vi "AlliGator Source Image Context Menu Handler.vi"(8 "Error In":errorcluster, 11 "Image Event Data":T3) -> (0 "Error Out":errorcluster, 3 "AlliGator Actions":T1[](array[typedef]))   [LabVIEW 2021, in "AlliGator Source Image.lvlib"]
doc: "Converts menu items into Source Image actions."
uses:
  AlliGator Source Image.lvlib
  Image/Image Display Event.ctl
  Image/Image Control Refnum.ctl
  <vilib>/Utility/miscctls.llb/LVPoint32TypeDef.ctl
  AlliGator Q Element.ctl
  AlliGator Q Event.ctl
  Image/Image Display to Clipboard Options.ctl
  AlliGator ROI Manager Actions.ctl
  AlliGator Selected ROI.ctl
  Image/Image Control ROI Description.ctl
  AlliGator Source Image ROI Manager.vi
  AlliGator Action Engine.lvlib
  Image/Image.lvlib
  Utilities/Utilities.lvlib
  AlliGator ROIs.lvlib
panel:
  # "see the AlliGator License on the block diagram (Ctrl+E or Window:Show Block Diagram)"
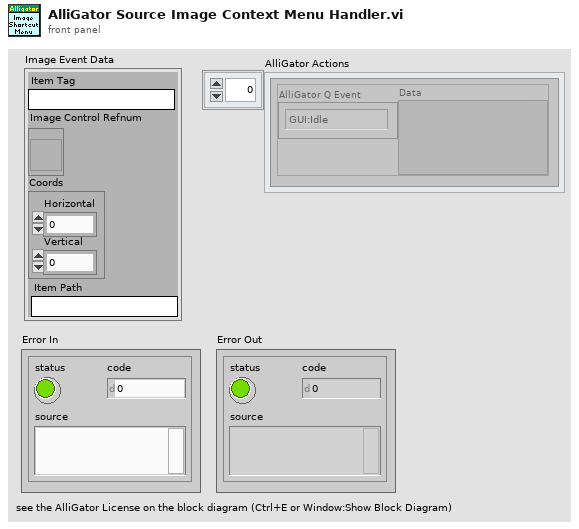
[diagram p1: front panel]
types:
  T1 = typedef "AlliGator Action Engine.lvlib/AlliGator Q Element.ctl" = cluster{"AlliGator Q Event":T2, "Data":variant}
  T2 = typedef "AlliGator Action Engine.lvlib/AlliGator Q Event.ctl" = enum16{"---- Files ----", "Files:Set Batch Export Files To Save", "Files:Set Dataset Loading & Pre-processing Options", "Files:Check #Frames in Dataset", "Files:Increment Frame Index", "Files:Open Mask Image", "Files:Open White Light Image", "Files:Open Single Dataset", "Files:New Folder of Folders Selected", "Files:Load File (all Types)_Scriptable", "Files:Move Flattened Series to Folders Series", "Files:Select Folder", "Files:Load FLI Dataset", "Files:Load Swiss SPAD 1 Dataset", "Files:Load Swiss SPAD 2 Dataset", "Files:Load .sdt FLI Dataset", "Files:Load .ptu FLI Dataset", "Files:Load .bin FLI Dataset", "Files:Load Single Gate Image Folder", "Files:Load I/m/phi Dataset (deprecated)", "Files:Load Single Image", "Files:Subtract Background File", "Files:Export FLI Dataset", "Files:Load HDF5 FLI Dataset", "Files:Set Destination File Path", "Files:Save Mask Image", "Files:Batch Conversion", "Files:New Folder Selected", "Files:Close FLI Dataset", "Files:Close FLI Dataset Series", "Files:Close White Light Image", "Files:Close Mask Image", "---- FLI Dataset ----", "FLI Dataset:Channel Arithmetic", "FLI Dataset:Export Average Lifetime Map as ASCII", "FLI Dataset:Export User-Defined Quantity Map as ASCII", "FLI Dataset:Python Function FLI Dataset Event", "FLI Dataset:ROI Analysis", "FLI Dataset:Tilted Logistic Square Gated IRF Characteristics Map", "FLI Dataset:Logistic Square Gated IRF Characteristics Map", "FLI Dataset:Square Gated IRF Characteristics Map", "FLI Dataset:Multi-ROI Single-Pixel Phasor Analysis", "FLI Dataset:Multi-ROI Single-Pixel NLSF Analysis", "FLI Dataset:All ROIs IRF Extraction", "FLI Dataset:All ROIs Decay Fit Non-Interactive (Fast + Individual IRF)", "FLI Dataset:All ROIs Phasor Analysis", "FLI Dataset:All ROIs Decay Fit", "FLI Dataset:Fluorescence Decay Statistics", "FLI Dataset:Update Decay Statistics Graph", "FLI Dataset:Get Decay from ROI", "FLI Dataset:All ROIs Average Lifetimes", "---- FLI Dataset Series ----", "FLI Dataset Series:Sum All Datasets in Series", "FLI Dataset Series:Add Dataset to Accumulated Dataset", "FLI Dataset Series:Display Accumulated Dataset", "FLI Dataset Series:Clear Dataset Series Sum", "FLI Dataset Series:Time-Series Analysis (NLSF)", "FLI Dataset Series:Time-Series Analysis (Phasor)", "---- Image ----", "Image:Update Image Profile Plots", "Image:Image Histogram Cursor Move", "Image:Image Histogram", "Image:Image Contrast", "Image:Set Image Histogram Cursor Move Flag", "Image:Clear Image Overlay", "Image:Use ROI as Search Area", "Image:Set ROI Diameter", "Image:Save Image Data as TIFF", "Image:Save Displayed Image with Overlay", "Image:Save Image Overlay Only", "Image:Save Image as Hot Pixel Mask", "Image:Change Source Image Color Palette", "Image:Copy Image to Clipboard", "Image:Source Image ROI Selection", "Image:Delete All ROIs", "Image:Delete All Unselected ROIs", "Image:Delete ROI", "Image:Merge All ROIs", "Image:Store ROI", "Image:Source Image ROI Storage", "Image:Export ROI Description to Notebook", "Image:Save ROI", "Image:Load ROI", "Image:Paste ROI Definition", "Image:Clear ROI", "Image:Identify ROIs in Mask Image", "Image:Create Complementary ROI", "Image:Create Contour ROI", "Image:Create ROI(s) from Pixels with Peak above Min_Scriptable", "Image:Create ROI(s) from Pixels with Intensity above Min_Scriptable", "Image:Compute ROI Statistics", "Image:Delete ROI(s) based on ROI Characteristics", "Image:Create ROI Grid", "Image:ROI to Individual Pixel ROIs", "Image:Python Function Source Image Event", "Image:Show Phasor Calibration Map ROI Centers", "Image:Convert ROI to Mask Image", "Image:Mouse Move", "Image:Mouse Up", "Image:Set Source Image Mouse Move Flag", "Image:Add Scale Bar Overlay", "Image:Delete Existing ROIs Option", "---- Decay ----", "Decay:Clear IRF/Reference Plot", "Decay:Clear Local IRFs", "Decay:Add Decay to Graph", "Decay:Smoothen Plot", "Decay:Smoothen Plot Tail", "Decay:Average Selected Plots", "Decay:Extract IRF", "Decay:Optimal IRF Extraction", "Decay:Threshold IRF", "Decay:Fit to Model IRF", "Decay:Fit IRF to Square Gate", "Decay:Fit IRF to Logistic Square Gate", "Decay:Fit IRF to Tilted Logistic Square Gate", "Decay:Create Bounding Cursors Set", "Decay:Export Bounding Cursors Definition to Notebook", "Decay:Denoise Plot", "Decay:Compute Cumulative Function", "Decay:Use as Reference Decay", "Decay:Show Reference Decay/IRF", "Decay:Extrapolate Decay", "Decay:Create Head & Tail Bounding Cursors", "Decay:Store Cursor-defined Head & Tail Fractions", "Decay:Rebin Plot", "Decay:1-Normalize Decay", "Decay:[0-1]-Normalize Plot", "Decay:Straighten Decay", "Decay:Shift Decay", "Decay:Fold Decay", "Decay:Fit Decay", "Decay:Global Fit of Selected Decays", "Decay:Post Global Fit Script", "Decay:Add Global Fit Parameters to Graph", "Decay:Add Decay Parameter(s) to Plot (Graph)", "Decay:Export Decay to Phasor Graph", "Decay:Plot Decay Shifts", "Decay:Compute Average Lifetime", "Decay:Plot Convolution", "Decay:Graph Tip Strip Update", "---- Decay Statistics ----", "Decay Statistics:Tip Strip Update", "---- Intensity Time Trace ----", "Intensity Time Trace:Use File Timestamp", "Intensity Time Trace:Load Intensity Corrections File", "Intensity Time Trace:Clear Intensity Corrections File", "Intensity Time Trace:Tip Strip Update", "---- Phasor Plot ----", "Phasor Plot:Build Phasor Plot", "Phasor Plot:Change Phasor Plot Color Palette", "Phasor Plot:Adjust Phasor Plot Display Range", "Phasor Plot:Highlight Image ROI in Phasor Plot", "Phasor Plot:Save Phasor Plot Image with Overlay", "Phasor Plot:Export Complex Phasor Map", "Phasor Plot:Export Phasor Ratio Map", "Phasor Plot:Export Average Lifetime Map", "Phasor Plot:Compute Phase Lifetime Histogram", "Phasor Plot:Compute Phasor Ratio Histogram", "Phasor Plot:Compute Phase Lifetime vs Intensity Scatter Plot", "Phasor Plot:Weber 2-Component Decomposition", "Phasor Plot:Update Phasor Color Map Vertices", "Phasor Plot:Clear Phasor Overlay", "Phasor Plot:Use Segment Extremities as References", "Phasor Plot:Use UC/Segment Intersections as References", "Phasor Plot:Use UC/Principal Axis Intersections as References", "Phasor Plot:Use UC/Linear Fit Intersections as References", "Phasor Plot:Update Phasor Plot Reference", "Phasor Plot:Show Local Phasor Info in Phasor Plot", "Phasor Plot:Update Phasor Plot State", "Phasor Plot:Phasor Plot ROI Storage", "Phasor Plot:Phasor Plot ROI Selection", "Phasor Plot:Python Function Phasor Plot Event", "Phasor Plot:Overlay Phasor ROI, Ratio or Map in Source Image", "Phasor Plot:Compute Decay of Selected Phasors", "Phasor Plot:Phasor at Image Pixel", "Phasor Plot:Mouse Move", "Phasor Plot:Mouse Up", "Phasor Plot:Display Range Mouse Move", "Phasor Plot:Set Mouse Move Flag", "---- Phasor Graph ----", "Phasor Graph:Calibrated Phasor Map Series", "Phasor Graph:Whole Image Phasor Scatter Plot (Todo)", "Phasor Graph:Get Phasor Value", "Phasor Graph:Create New Phasor Plot Dialog", "Phasor Graph:Update Last Phasor Value", "Phasor Graph:Update Phasor (m, phi)", "Phasor Graph:Remove Single Phasor from Plot", "Phasor Graph:Add Single Phasor to Plot", "Phasor Graph:Remove Phasor Plot", "Phasor Graph:Remove Selected Phasor Plots", "Phasor Graph:Clear Phasor Data", "Phasor Graph:Clear Phasor Graph", "Phasor Graph:Cursor Move", "Phasor Graph:Draw Cursor Connecting Line", "Phasor Graph:Clear Cursor Connecting Line", "Phasor Graph:Find UC Intersection", "Phasor Graph:Use UC/Cursor-Defined Line Intersections", "Phasor Graph:Use Selected Plots Fitted Line/UC Intersections", "Phasor Graph:Use Selected Plots Principal Axis/UC Intersections", "Phasor Graph:Show Single Phasor", "Phasor Graph:Save Single Phasor Plot", "Phasor Graph:Save All Phasor Plots", "Phasor Graph:Load Phasor Plot(s)", "Phasor Graph:Phasor Multiplication", "Phasor Graph:Compute Average Phasor", "Phasor Graph:Compute Multiple Average Phasors (Selected Plots)", "Phasor Graph:Export Single Phasor Plot Phase Lifetimes", "Phasor Graph:Phase Lifetime Trajectory", "Phasor Graph:Phase Lifetime vs Intensity Scatter Plot (deprecated)", "Phasor Graph:Parameter 2 vs Parameter 1 Scatter Plot", "Phasor Graph:Use Cursor n Location", "Phasor Graph:Set Reference n to Current Phase Lifetime Value", "Phasor Graph:Set Reference n to Lifetime Value", "Phasor Graph:Set Cursor n Location", "Phasor Graph:Save Phasor Graph Image", "Phasor Graph:Update SEPL Plot", "Phasor Graph:Export Single Phasor Plot Data", "Phasor Graph:Export Selected Phasor Plots Data", "Phasor Graph:Python Function Phasor Graph Event", "Phasor Graph:Tip Strip Update", "---- Calibration ----", "Calibration:Set Calibration Type", "Calibration:Load/Save Phasor Calibration", "Calibration:Load/Save Phasor Calibration Series", "Calibration:Load/Save Phasor Calibration Map", "Calibration:Use as Calibration", "Calibration:Compute Optimal Calibration from Phasor References", "Calibration:Clear Phasor Calibration", "Calibration:Use as Calibration Series", "Calibration:Use as Calibration Map", "Calibration:Clear Calibration Series", "Calibration:Clear Calibration Map", "Calibration:Apply Phasor Calibration", "Calibration:Update Single Plot Calibration", "Calibration:Update Multiple Plots Calibration", "Calibration:Clear Single Plot Calibration", "Calibration:Clear All Plots Calibrations", "Calibration:Clear Plot(s) Calibration(s)?", "Calibration:Phasor Calibration Maps (# Gates Series)", "---- Phasor Ratio ----", "Phasor Ratio:Clear Reference n", "Phasor Ratio:Toggle Selected Plot(s)  Lock to Reference 1", "Phasor Ratio:Use as Reference n", "Phasor Ratio:Send Reference n to Notebook", "Phasor Ratio:Toggle Selected Plot(s)  Lock to Reference 2", "Phasor Ratio:Compute Phasor Ratio at Mouse Location", "Phasor Ratio:Compute Phasor Plot's Average Phasor Ratio", "Phasor Ratio:Compute Time-Series Phasor Ratios", "Phasor Ratio:Fit Line to Phasor Ratio Plot", "Phasor Ratio:Save References", "Phasor Ratio:Load References", "Phasor Ratio:Update Phasor Reference 1", "Phasor Ratio:Update Phasor Reference 2", "Phasor Ratio:Move Cursor n to Reference n", "Phasor Ratio:Use as Phasor Reference 1 Lifetime", "Phasor Ratio:Use as Phasor Reference 2 Lifetime", "Phasor Ratio:Export Phasor Ratio Map as ASCII", "Phasor Ratio:Tip Strip Update", "---- Lifetime & Other Parameters Graph ----", "Lifetime:Tip Strip Update", "---- Decay Fit Parameter Map ----", "Decay Fit Parameter Map:Export ROI NLSF Data as ASCII", "Decay Fit Parameter Map:Set Decay Fit  Parameter Map Selection", "Decay Fit Parameter Map:Build Decay Fit Parameter Map", "Decay Fit Parameter Map:Change Decay Fit Parameter Map Color Palette", "Decay Fit Parameter Map:Export Decay Fit Parameter Map Data as ASCII", "Decay Fit Parameter Map:Export All Decay Fit Parameter Maps Data as ASCII", "Decay Fit Parameter Map:Send Map Data to Lifetime Graph", "Decay Fit Parameter Map:Save Decay Fit Parameter Map Image", "Decay Fit Parameter Map:Save-Load IRFs & Fit Data", "Decay Fit Parameter Map:Update Local Decay Plots", "Decay Fit Parameter Map:Python Function Decay Fit Parameters Map Event", "Decay Fit Parameter Map:Overlay Decay Fit Parameter Map in Source Image", "Decay Fit Parameter Map:Plot Map Data vs Intensity", "Decay Fit Parameter Map:Mouse Up", "Decay Fit Parameter Map:Display Range Mouse Move", "---- Generic Graph ----", "Generic Graph:Generic XY Graph Event", "Generic Graph:Python Function XY Graph Event", "Generic Graph:New Plot", "Generic Graph:Save Plot", "Generic Graph:XY Plot Histogram", "Generic Graph:Set XY Graph Plot Name", "Generic Graph:Set Last Cursor Style", "Generic Graph:Tip Strip Update", "---- GUI ----", "GUI:Start Script", "GUI:Type of Displayed Image Changed", "GUI:Gate Image Slide Changed", "GUI:Show Busy Icon", "GUI:Show Busy Icon & Abort Button", "GUI:Hide Busy Icon", "GUI:Hide Busy Icon & Abort Button", "GUI:Abort", "GUI:End Script", "GUI:Start Timing", "GUI:End Timing", "GUI:Set State Indicator", "GUI:Send Parameters JSON Strings to Clipboard", "GUI:Set Gate Step", "GUI:Idle", "GUI:Initialization", "GUI:Quit", "GUI:Increment Dataset Index", "GUI:Set Dataset Index to -1", "GUI:Time Series Slider Moved", "GUI:Time Series Slider Changed", "GUI:Toggle Playback or Loop", "GUI:Playback Script", "GUI:Set Phasor Frequency", "GUI:Open Window", "DEBUG"}
  T3 = typedef "Image.lvlib/Image Display Event.ctl" = cluster{"Item Tag":string, "Image Control Refnum":T4, "Coords":T5, "Item Path":string}
  T4 = typedef "Image.lvlib/Image Control Refnum.ctl" = refnum<vi>
  T5 = typedef "LVPoint32TypeDef.ctl" = cluster{"Horizontal":i32, "Vertical":i32}
  T6 = typedef "Image.lvlib/Image Display to Clipboard Options.ctl" = cluster{"Include Overlay (T)":bool, "Image Only (T)":bool}
  T7 = typedef "AlliGator ROIs.lvlib/AlliGator ROI Manager Actions.ctl" = enum16{"Undefined", "Delete Current ROI", "Delete All Unselected ROIs", "Delete Multiple ROIs", "Delete All ROIs", "Swap ROIs", "Insert ROI", "Update Current ROI Descriptor", "Rename Current ROI", "Store New ROI", "Store Multiple ROIs", "Select Next ROI", "Select Previous ROI", "Find Selected ROI", "Show All ROIs", "Update ROI Manager Window", "Merge All ROIs", "Unmerge ROI", "Set Selected ROI by ID"}
  T8 = typedef "AlliGator ROIs.lvlib/AlliGator Selected ROI.ctl" = cluster{"Image Ctrl Ref":T4, "All ROIs?":bool}
  T9 = typedef "Image.lvlib/Image Control ROI Description.ctl" = cluster{"Image Control Label":string, "ROI Descriptor":T10}
  T10 = typedef "ROI Descriptor" = cluster{"Global Rectangle":i32[], "Contours":cluster{"ID":enum32{"External", "Internal"}, "Type":u32, "Coordinates":i32[]}[]}
  T11 = cluster{"Image Control Refnum":T4, "Image to Clipboard Options":T6}
  T12 = cluster{"Global Rectangle":i32[], "Contours":cluster{"Contour Type":u32, "ROI Type":u32, "Points":i32[]}[]}
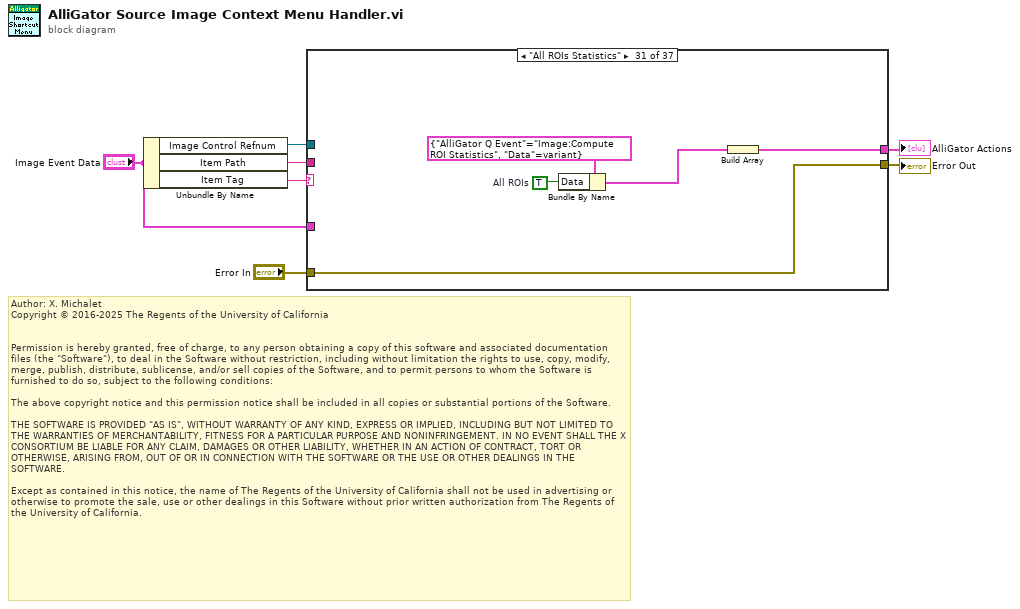
[diagram p0: block diagram]
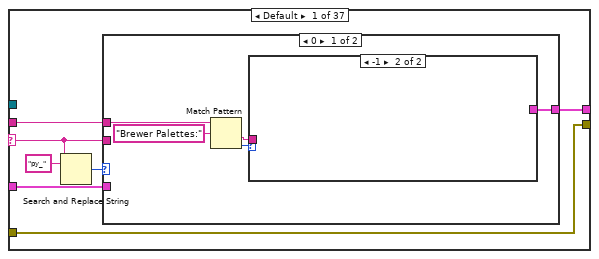
[diagram p2: hidden frame]
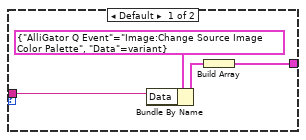
[diagram p3: hidden frame]
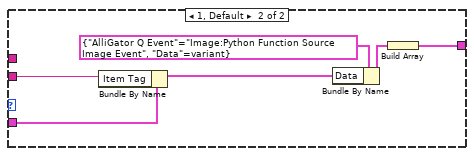
[diagram p4: hidden frame]
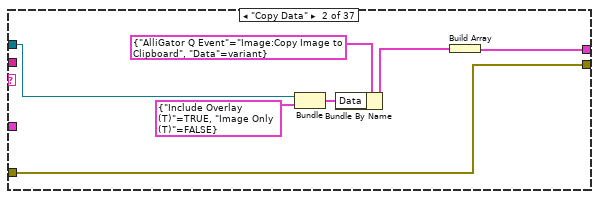
[diagram p5: hidden frame]
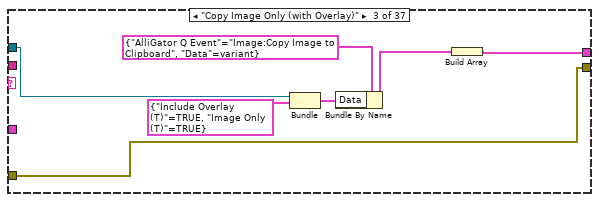
[diagram p6: hidden frame]
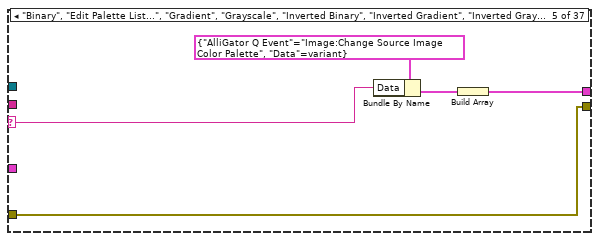
[diagram p8: hidden frame]
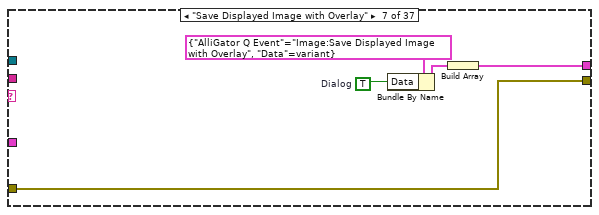
[diagram p10: hidden frame]
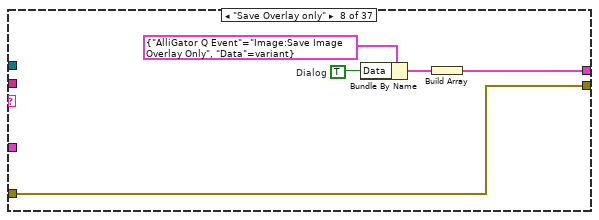
[diagram p11: hidden frame]
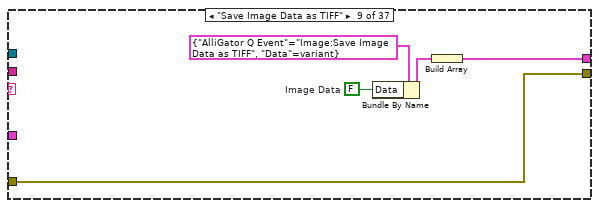
[diagram p12: hidden frame]
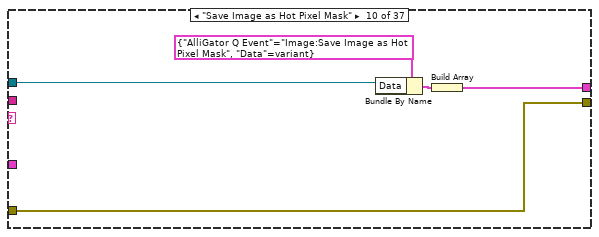
[diagram p13: hidden frame]
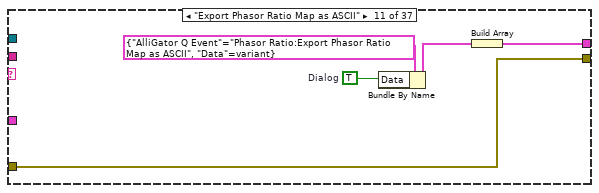
[diagram p14: hidden frame]
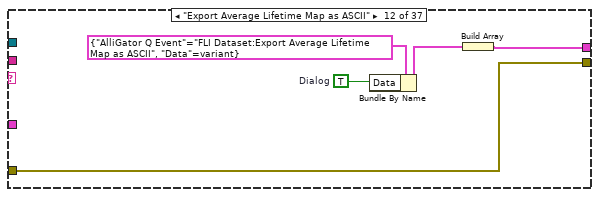
[diagram p15: hidden frame]
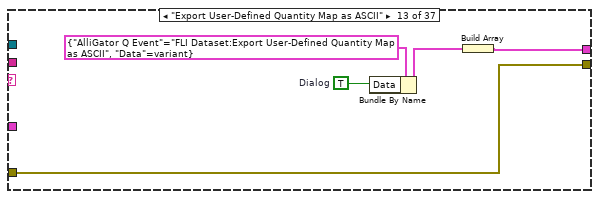
[diagram p16: hidden frame]
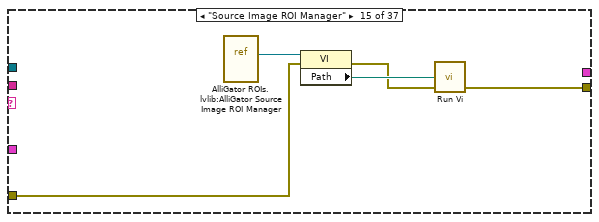
[diagram p18: hidden frame]
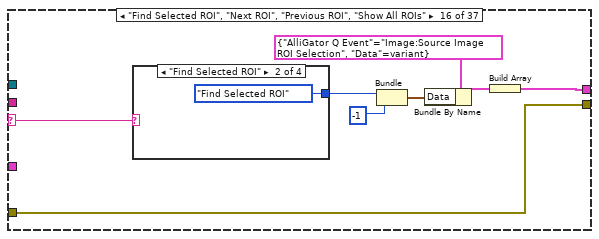
[diagram p19: hidden frame]
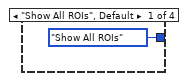
[diagram p20: hidden frame]
diagram:
  # "Author: X. Michalet\nCopyright © 2016-2025 The Regents of the University of California\n \n\nPermission is hereby granted, free of charge, to any person obtaining a copy of this software and associated documentation files (the \"Software\"), to deal in the Software without restriction, including without limitation the rights to use, copy, modify, merge, publish, distribute, sublicense, and/or sell copies of the Software, and to permit persons to whom the Software is furnished to do so, subject to the following conditions:\n\nThe above copyright notice and this permission notice shall be included in all copies or substantial portions of the Software.\n\nTHE SOFTWARE IS PROVIDED \"AS IS\", WITHOUT WARRANTY OF ANY KIND, EXPRESS OR IMPLIED, INCLUDING BUT NOT LIMITED TO THE WARRANTIES OF MERCHANTABILITY, FITNESS FOR A PARTICULAR PURPOSE AND NONINFRINGEMENT. IN NO EVENT SHALL THE X CONSORTIUM BE LIABLE FOR ANY CLAIM, DAMAGES OR OTHER LIABILITY, WHETHER IN AN ACTION OF CONTRACT, TORT OR OTHERWISE, ARISING FROM, OUT OF OR IN CONNECTION WITH THE SOFTWARE OR THE USE OR OTHER DEALINGS IN THE SOFTWARE.\n\nExcept as contained in this notice, the name of The Regents of the University of California shall not be used in advertising or otherwise to promote the sale, use or other dealings in this Software without prior written authorization from The Regents of the University of California."
  n1 = Unbundle By Name("Image Event Data") -> ("Image Control Refnum"=w5:T4, "Item Path"=w4:string, "Item Tag"=w3:string)
  n2 = case shown="\"All ROIs Statistics\"" w3 {
    selector: w3 -> [w8 _ _ _ w47 _ _ _ _ _ _ _ _ _ _ w95 _ w111 _ _ _ _ _ _ _ _ _ _ _ _ _ _ _ _ _ _ _]
    tunnel: w5 -> [_ w32 w39 _ _ _ _ _ _ w66 _ _ _ _ _ _ w107 _ _ w129 w135 w142 _ _ _ _ _ _ _ _ _ _ _ w187 _ w192 w194]
    tunnel: w4 -> [w14 _ _ _ _ _ _ _ _ _ _ _ _ _ _ _ _ _ _ _ _ _ _ _ _ _ _ _ _ _ _ _ _ _ _ _ _]
    tunnel: [w13 w31 w38 _ w46 _ w52 w58 w63 w68 w71 w76 w81 _ _ w97 w105 w113 T1[] [{"AlliGator Q Event"=enum."Image:Delete ROI(s) based on ROI Characteristics", "Data"=variant}] ("element") w125 w133 w141 T1[] [{"AlliGator Q Event"=enum."Image:Paste ROI Definition", "Data"=variant}] ("element") T1[] [{"AlliGator Q Event"=enum."Image:Create Complementary ROI", "Data"=variant}] ("element") T1[] [{"AlliGator Q Event"=enum."Image:Create Contour ROI", "Data"=variant}] ("element") T1[] [{"AlliGator Q Event"=enum."Image:Create ROI(s) from Pixels with Peak above Min_Scriptable", "Data"=variant}] ("element") T1[] [{"AlliGator Q Event"=enum."Image:Create ROI(s) from Pixels with Intensity above Min_Scriptable", "Data"=variant}] ("element") T1[] [{"AlliGator Q Event"=enum."Image:Create ROI Grid", "Data"=variant}] ("element") T1[] [{"AlliGator Q Event"=enum."Image:ROI to Individual Pixel ROIs", "Data"=variant}] ("element") w160 w165 w170 w175 w181 _ _ _] -> w1
    tunnel: "Error In" -> [w12 w30 w37 w44 w45 w50 w55 w57 w62 w67 w75 w80 w85 w86 w88 w96 w104 w112 w123 w124 w132 w140 w145 w147 w149 w151 w153 w155 w157 w163 w168 w173 w178 w179 w189 w190 w193]
    tunnel: [w12 w30 w37 w44 w45 w50 w55 w57 w62 w67 w75 w80 w85 w86 w87 w96 w104 w112 w123 w124 w132 w140 w145 w147 w149 w151 w153 w155 w157 w163 w168 w173 w178 w180 w189 w190 w193] -> w6
    tunnel: "Image Event Data" -> [w9 _ _ _ _ _ _ _ _ _ _ _ _ _ _ _ _ _ _ _ _ _ _ _ _ _ _ _ _ _ _ _ _ _ _ _ _]
    frame Default {
      n3 = Search and Replace String(input string=w8, search string="py_") -> (number of replacements=w10:i32)  [unwired: 6 in, 3 out]
      n4 = case shown="0" w10 {
        tunnel: w14 -> [w19 _]
        tunnel: [w15 w28] -> w13
        tunnel: w8 -> [_ w24]
        tunnel: w9 -> [_ w26]
        frame 0 {
          n5 = Match Pattern(string=w19, regular expression="Brewer Palettes:") -> (after substring=w16:string, offset past match=w17:i32)  [unwired: 1 in, 2 out]
          n6 = case shown="-1" w17 {
            tunnel: w16 -> [w21 _]
            tunnel: [w20 _] -> w15
            frame Default {
              n7 = Bundle By Name(cluster=T1 {"AlliGator Q Event"=enum."Image:Change Source Image Color Palette", "Data"=variant} ("element"), "Data"=w21) -> (w22:T1)
              n8 = Build Array(w22) -> (w20:T1[])
            }
            frame -1 {
            }
          }
        }
        frame 1, Default {
          n9 = Bundle By Name(cluster=w26, "Item Tag"=w24) -> (w25:T3)
          n10 = Bundle By Name(cluster=T1 {"AlliGator Q Event"=enum."Image:Python Function Source Image Event", "Data"=variant}, "Data"=w25) -> (w27:T1)
          n11 = Build Array(w27) -> (w28:T1[])
        }
      }
    }
    frame "Copy Data" {
      n12 = Bundle("Image Control Refnum"=w32, "Image to Clipboard Options"=T6 {"Include Overlay (T)"=TRUE, "Image Only (T)"=FALSE}) -> (w33:T11)  [unwired: 1 in]
      n13 = Bundle By Name(cluster=T1 {"AlliGator Q Event"=enum."Image:Copy Image to Clipboard", "Data"=variant} ("element"), "Data"=w33) -> (w35:T1)
      n14 = Build Array(w35) -> (w31:T1[])
    }
    frame "Copy Image Only (with Overlay)" {
      n15 = Bundle("Image Control Refnum"=w39, "Image to Clipboard Options"=T6 {"Include Overlay (T)"=TRUE, "Image Only (T)"=TRUE}) -> (w40:T11)  [unwired: 1 in]
      n16 = Bundle By Name(cluster=T1 {"AlliGator Q Event"=enum."Image:Copy Image to Clipboard", "Data"=variant} ("element"), "Data"=w40) -> (w42:T1)
      n17 = Build Array(w42) -> (w38:T1[])
    }
    frame "---------Palette----------" {
    }
    frame "Binary", "Edit Palette List...", "Gradient", "Grayscale", "Inverted Binary", "Inverted Gradient", "Inverted Grayscale", "Inverted Rainbow", "Inverted Temperature", "Rainbow", "Select New Palette...", "Temperature" {
      n18 = Bundle By Name(cluster=T1 {"AlliGator Q Event"=enum."Image:Change Source Image Color Palette", "Data"=variant} ("element"), "Data"=w47) -> (w48:T1)
      n19 = Build Array(w48) -> (w46:T1[])
    }
    frame "--------- Others  ---------" {
    }
    frame "Save Displayed Image with Overlay" {
      w51 = TRUE  # Dialog
      n20 = Bundle By Name(cluster=T1 {"AlliGator Q Event"=enum."Image:Save Displayed Image with Overlay", "Data"=variant} ("Time-Gated Phasor Q Element"), "Data"=w51) -> (w53:T1)
      n21 = Build Array(w53) -> (w52:T1[])
    }
    frame "Save Overlay only" {
      w56 = TRUE  # Dialog
      n22 = Bundle By Name(cluster=T1 {"AlliGator Q Event"=enum."Image:Save Image Overlay Only", "Data"=variant} ("element"), "Data"=w56) -> (w59:T1)
      n23 = Build Array(w59) -> (w58:T1[])
    }
    frame "Save Image Data as TIFF" {
      w61 = FALSE  # Image Data
      n24 = Bundle By Name(cluster=T1 {"AlliGator Q Event"=enum."Image:Save Image Data as TIFF", "Data"=variant} ("element"), "Data"=w61) -> (w64:T1)
      n25 = Build Array(w64) -> (w63:T1[])
    }
    frame "Save Image as Hot Pixel Mask" {
      n26 = Bundle By Name(cluster=T1 {"AlliGator Q Event"=enum."Image:Save Image as Hot Pixel Mask", "Data"=variant} ("element"), "Data"=w66) -> (w69:T1)
      n27 = Build Array(w69) -> (w68:T1[])
    }
    frame "Export Phasor Ratio Map as ASCII" {
      w72 = TRUE  # Dialog
      n28 = Bundle By Name(cluster=T1 {"AlliGator Q Event"=enum."Phasor Ratio:Export Phasor Ratio Map as ASCII", "Data"=variant} ("element"), "Data"=w72) -> (w73:T1)
      n29 = Build Array(w73) -> (w71:T1[])
    }
    frame "Export Average Lifetime Map as ASCII" {
      w77 = TRUE  # Dialog
      n30 = Bundle By Name(cluster=T1 {"AlliGator Q Event"=enum."FLI Dataset:Export Average Lifetime Map as ASCII", "Data"=variant} ("element"), "Data"=w77) -> (w78:T1)
      n31 = Build Array(w78) -> (w76:T1[])
    }
    frame "Export User-Defined Quantity Map as ASCII" {
      w82 = TRUE  # Dialog
      n32 = Bundle By Name(cluster=T1 {"AlliGator Q Event"=enum."FLI Dataset:Export User-Defined Quantity Map as ASCII", "Data"=variant} ("element"), "Data"=w82) -> (w83:T1)
      n33 = Build Array(w83) -> (w81:T1[])
    }
    frame "------ ROIs ------" {
    }
    frame "Source Image ROI Manager" {
      n34 = vi-ref "AlliGator ROIs.lvlib:AlliGator Source Image ROI Manager.vi"() -> (w91:refnum<vi>)
      n35 = property class="VI"(reference=w91, error in=w88) -> (error out=w89:errorcluster, "Path"=w90:path)  [unwired: 1 out]
      n36 = call "Run Vi.vi"("VI Path"=w90, "error in (no error)"=w89) -> ("error out"=w87:errorcluster)  [unwired: 6 in, 1 out]
    }
    frame "Find Selected ROI", "Next ROI", "Previous ROI", "Show All ROIs" {
      n37 = case shown="\"Find Selected ROI\"" w95 {
        tunnel: [AlliGator_ROI_Manager_Actions."Show All ROIs" ("Action") AlliGator_ROI_Manager_Actions."Find Selected ROI" ("Action") AlliGator_ROI_Manager_Actions."Select Next ROI" ("Action") AlliGator_ROI_Manager_Actions."Select Previous ROI" ("Action")] -> w93
        frame "Show All ROIs", Default {
        }
        frame "Find Selected ROI" {
        }
        frame "Next ROI" {
        }
        frame "Previous ROI" {
        }
      }
      n38 = Bundle("Action"=w93, -1) -> (w92:cluster{"Action":T7, i32})  [unwired: 1 in]
      n39 = Bundle By Name(cluster=T1 {"AlliGator Q Event"=enum."Image:Source Image ROI Selection", "Data"=variant} ("element"), "Data"=w92) -> (w98:T1)
      n40 = Build Array(w98) -> (w97:T1[])
    }
    frame "Hide All ROIs" {
      n41 = property class="ImageControl"(reference=w107) -> ("Label.Text"=w106:string)  [unwired: 1 in, 2 out]
      n42 = Bundle By Name(cluster=T1 {"AlliGator Q Event"=enum."Image:Clear ROI", "Data"=variant} ("element"), "Data"=w106) -> (w108:T1)
      n43 = Build Array(w108) -> (w105:T1[])
    }
    frame "Delete All ROIs", "Delete All Unselected ROIs", "Delete ROI", "Merge All ROIs", "Store ROI" {
      n44 = case shown="\"Store ROI\"" w111 {
        tunnel: [AlliGator_ROI_Manager_Actions."Delete Current ROI" ("Action") AlliGator_ROI_Manager_Actions."Delete All Unselected ROIs" ("Action") AlliGator_ROI_Manager_Actions."Delete All ROIs" ("Action") AlliGator_ROI_Manager_Actions."Store New ROI" ("Action") AlliGator_ROI_Manager_Actions."Merge All ROIs" ("Action") AlliGator_ROI_Manager_Actions."Unmerge ROI" ("Action")] -> w110
        frame "Delete ROI", Default {
        }
        frame "Delete All Unselected ROIs" {
        }
        frame "Delete All ROIs" {
        }
        frame "Store ROI" {
        }
        frame "Merge All ROIs" {
        }
        frame "Unmerge ROI" {
        }
      }
      n45 = Bundle By Name(cluster=T1 {"AlliGator Q Event"=enum."Image:Source Image ROI Storage", "Data"=variant} ("element"), "Data"=w110) -> (w114:T1)
      n46 = Build Array(w114) -> (w113:T1[])
    }
    frame "Delete ROI(s) based on ROI Characteristics" {
    }
    frame "Save Current ROI" {
      n47 = Bundle(cluster=T8 {"Image Ctrl Ref"=refnum, "All ROIs?"=TRUE} ("Selected ROI"), "Image Ctrl Ref"=w129, "All ROIs?"=FALSE) -> (w127:T8)
      n48 = Bundle By Name(cluster=T1 {"AlliGator Q Event"=enum."Image:Save ROI", "Data"=variant} ("element"), "Data"=w127) -> (w130:T1)
      n49 = Build Array(w130) -> (w125:T1[])
    }
    frame "Save All ROIs" {
      n50 = Bundle(cluster=T8 {"Image Ctrl Ref"=refnum, "All ROIs?"=TRUE} ("Selected ROI"), "Image Ctrl Ref"=w135, "All ROIs?"=TRUE) -> (w136:T8)
      n51 = Bundle By Name(cluster=T1 {"AlliGator Q Event"=enum."Image:Save ROI", "Data"=variant} ("element"), "Data"=w136) -> (w138:T1)
      n52 = Build Array(w138) -> (w133:T1[])
    }
    frame "Load ROI(s)" {
      n53 = Bundle By Name(cluster=T1 {"AlliGator Q Event"=enum."Image:Load ROI", "Data"=variant} ("element"), "Data"=w142) -> (w143:T1)
      n54 = Build Array(w143) -> (w141:T1[])
    }
    frame "Paste ROI Definition" {
    }
    frame "Create Complementary ROI" {
    }
    frame "Create Contour ROI (deprecated)" {
    }
    frame "Create ROI(s) from Pixels with Peak above Min" {
    }
    frame "Create ROI(s) from Pixels with Intensity above Min" {
    }
    frame "Create ROI Grid" {
    }
    frame "ROI to Individual Pixel ROIs" {
    }
    frame "Curent ROI Characteristics", "Current ROI Statistics" {
      w159 = FALSE  # Current ROI
      n55 = Bundle By Name(cluster=T1 {"AlliGator Q Event"=enum."Image:Compute ROI Statistics", "Data"=variant} ("Time-Gated Phasor Q Element"), "Data"=w159) -> (w161:T1)
      n56 = Build Array(w161) -> (w160:T1[])
    }
    frame "All ROIs Statistics" {
      w164 = TRUE  # All ROIs
      n57 = Bundle By Name(cluster=T1 {"AlliGator Q Event"=enum."Image:Compute ROI Statistics", "Data"=variant} ("Time-Gated Phasor Q Element"), "Data"=w164) -> (w166:T1)
      n58 = Build Array(w166) -> (w165:T1[])
    }
    frame "Convert ROI to Mask Image" {
      w169 = FALSE  # Selected ROI
      n59 = Bundle By Name(cluster=T1 {"AlliGator Q Event"=enum."Image:Convert ROI to Mask Image", "Data"=variant} ("Time-Gated Phasor Q Element"), "Data"=w169) -> (w171:T1)
      n60 = Build Array(w171) -> (w170:T1[])
    }
    frame "Convert All ROIs to Mask Image" {
      w174 = TRUE  # All ROIs
      n61 = Bundle By Name(cluster=T1 {"AlliGator Q Event"=enum."Image:Convert ROI to Mask Image", "Data"=variant} ("Time-Gated Phasor Q Element"), "Data"=w174) -> (w176:T1)
      n62 = Build Array(w176) -> (w175:T1[])
    }
    frame "Export ROI Description to Notebook" {
      n63 = property class="ImageControl"(reference=w187, error in=w179) -> (error out=w180:errorcluster, "Label.Text"=w185:string, "ROI"=w184:T12)  [unwired: 1 out]
      n64 = Bundle By Name(cluster=T9 {"Image Control Label"="", "ROI Descriptor"={"Global Rectangle"=[], "Contours"=[]}}, "Image Control Label"=w185, "ROI Descriptor"=w184) -> (w182:T9)
      n65 = Bundle By Name(cluster=T1 {"AlliGator Q Event"=enum."Image:Export ROI Description to Notebook", "Data"=variant} ("element"), "Data"=w182) -> (w186:T1)
      n66 = Build Array(w186) -> (w181:T1[])
    }
    frame "--------------" {
    }
    frame "Zoom to Fit" {
      n67 = call "Image Display Zoom to Fit.vi"("Keep Aspect Ratio (T)"=FALSE, "Display Image Control Refnum"=w192) -> ()  [unwired: 9 in, 1 out]
    }
    frame "Zoom to Fit (Keep Aspect Ratio)" {
      n68 = call "Image Display Zoom to Fit.vi"("Display Image Control Refnum"=w194) -> ()  [unwired: 10 in, 1 out]
    }
  }
  "Error Out" <- w6
  "AlliGator Actions" <- w1
